vi "Project Spec Type.vi"(0 "NI Build Specification in":refnum<class "NI Build Specification_LV.lvclass">, 11 "error in (no error)":errorcluster) -> (4 "NI Build Specification out":refnum<class "NI Build Specification_LV.lvclass">, 6 "Project Specfication Type":string, 15 "error out":errorcluster)   [LabVIEW 2017, in "CL_G3_VIComponentBuilder.lvlib" / "NI Build Specification_LV.lvclass"]
doc: "Returns the type of spec as defined by NI.\n<RequiredOverrideReason>Each build spec type has its own unique type string which must be defined.</RequiredOverrideReason>"
uses:
  NI Build Specification_LV.lvclass
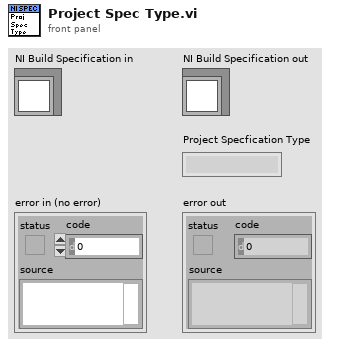
[diagram p1: front panel]
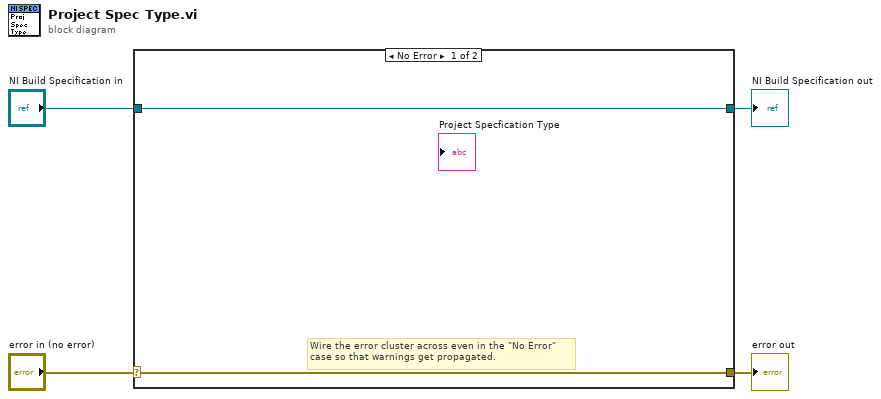
[diagram p0: block diagram]
diagram:
  n1 = case shown="No Error" "error in (no error)" {
    selector: "error in (no error)" -> [w5 w8]
    tunnel: [w5 w8] -> w3
    tunnel: [w6 w7] -> w1
    tunnel: "NI Build Specification in" -> [w6 w7]
    frame No Error {
      # "Wire the error cluster across even in the \"No Error\"\ncase so that warnings get propagated."
    }
    frame Error {
    }
  }
  "error out" <- w3
  "NI Build Specification out" <- w1
